vi "GlobalFGVVI.vi"() -> ()   [LabVIEW 2017]
panel:
  out "Final value":i32
  in  "stop":bool
  in  "Starting value":i32
  out "Sum":i32
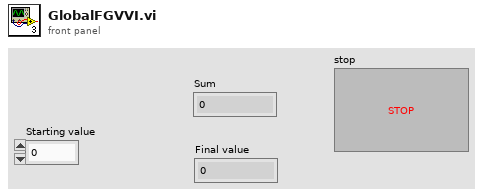
[diagram p1: front panel]
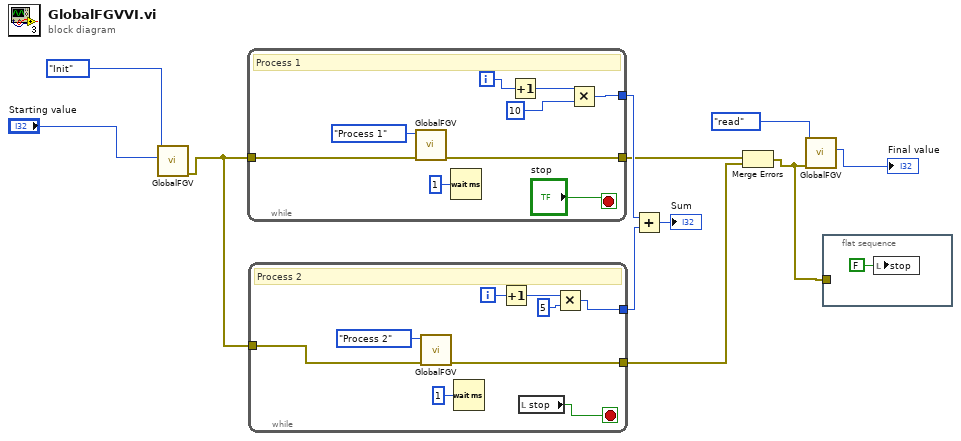
[diagram p0: block diagram]
diagram:
  n1 = call "GlobalFGV.vi"("Initial position"="Starting value", "Enum"=enum16{"Process 2", "Process 1", "Init", "read"}."Init") -> ("error out"=w6:errorcluster)  [unwired: 8 in, 1 out]
  n2 = while {
    tunnel: [w18] -> w11
    tunnel: w6 -> [w14]
    tunnel: [w12] -> w5
    i -> [w19]
    stop <- "stop" stop-if-true
    # "Process 1"
    n3 = call "GlobalFGV.vi"("error in (no error)"=w14, "Enum"=enum16{"Process 2", "Process 1", "Init", "read"}."Process 1") -> ("error out"=w12:errorcluster)  [unwired: 8 in, 1 out]
    n4 = Wait (ms)(milliseconds to wait=u32 1) -> ()  [unwired: 1 out]
    n5 = Increment(x=w19) -> (x+1=w20:i32)
    n6 = Multiply(x=w20, y=10) -> (x*y=w18:i32)
  }
  n7 = while {
    tunnel: [w26] -> w9
    tunnel: w6 -> [w23]
    tunnel: [w21] -> w4
    i -> [w28]
    stop <- w24 stop-if-true
    # "Process 2"
    n8 = call "GlobalFGV.vi"("error in (no error)"=w23, "Enum"=enum16{"Process 2", "Process 1", "Init", "read"}."Process 2") -> ("error out"=w21:errorcluster)  [unwired: 8 in, 1 out]
    n9 = Wait (ms)(milliseconds to wait=u32 1) -> ()  [unwired: 1 out]
    n10 = Increment(x=w28) -> (x+1=w29:i32)
    n11 = local read "stop"() -> (w24:bool)
    n12 = Multiply(x=w29, y=5) -> (x*y=w26:i32)
  }
  n13 = Add(x=w11, y=w9) -> (x+y=→"Sum":i32)
  n14 = Merge Errors(w5, w4) -> (w1:errorcluster)
  n15 = call "GlobalFGV.vi"("error in (no error)"=w1, "Enum"=enum16{"Process 2", "Process 1", "Init", "read"}."read") -> ("New position"=→"Final value":i32)  [unwired: 8 in, 1 out]
  n16 = flat-sequence {
    tunnel: w1 -> [_]
    frame #0 {
      n17 = local write "stop"(FALSE ("stop")) -> ()
    }
  }
